vi "CLSUIP_GetReplaceArrSubsetNode.vi"(8 "error in (no error)":errorcluster, 11 "VI Refnum":refnum<vi>) -> (0 "error out":errorcluster, 2 "ReplaceArraySubset Node Ref":refnum<vi>, 3 "VI Refnum out":refnum<vi>)   [LabVIEW 2021, in "MemberVICreation.lvlib"]
uses:
  <resource>/Framework/Providers/LVClassLibrary/NewAccessors/MemberVICreation.lvlib
  <vilib>/Utility/traverseref.llb/TRef TravTarget.ctl
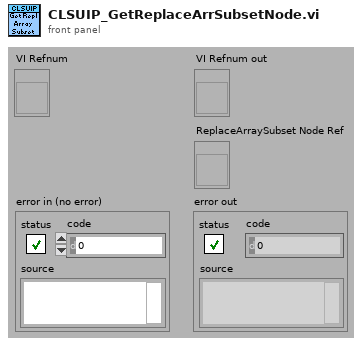
[diagram p1: front panel]
types:
  T1 = typedef "TRef TravTarget.ctl" = enum16{"FP", "BD", "Other"}
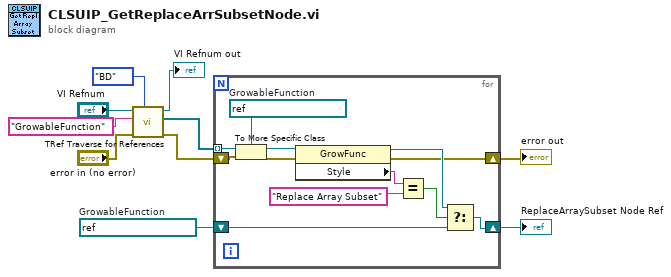
[diagram p0: block diagram]
diagram:
  w3 = refnum<vi> refnum  # GrowableFunction
  n1 = call <vilib>:"TRef Traverse for References.vi"("Traverse Target"=TRef_TravTarget."BD", "error in (no error)"="error in (no error)", "Class Name"="GrowableFunction" ("y"), "VI Refnum"="VI Refnum") -> ("error out"=w4:errorcluster, "References"=w5:refnum<vi>[], "dup VI Refnum"=→"VI Refnum out":refnum<vi>)  [unwired: 1 in, 4 out]
  n2 = for {
    tunnel: w5 -> [w22] mode=indexing
    shift-right: [w11] -> w1
    shift-left: w4 -> [w20]
    shift-right: [w13] -> w2
    shift-left: w3 -> [w14]
    w21 = refnum<vi> refnum  # GrowableFunction
    n3 = To More Specific Class(target class=w21, reference=w22, error in=w20) -> (specific class reference=w19:refnum<vi>, error out=w18:errorcluster)
    n4 = property class="GrowFunc"(reference=w19, error in=w18) -> (reference out=w12:refnum<vi>, error out=w11:errorcluster, "Style"=w17:string)
    n5 = Equal?(x=w17, y="Replace Array Subset") -> (x = y?=w15:bool)
    n6 = Select(t=w12, s=w15, f=w14) -> (s? t:f=w13:refnum<vi>)
  }
  "error out" <- w1
  "ReplaceArraySubset Node Ref" <- w2
